vi "SDCP SMF Receiver and Transmitter - Read Processed Trace File.vi"(3 "error in (no error)":errorcluster, 4 "Trace File Path":path=path "E:/Projects/System Diagnostics and Control Protocol/SDCP_LabVIEW/temp/Trace Files/21 Apr 2024 20-17.csv", 5 "Parameter file path":path=path "E:/Projects/System Diagnostics and Control Protocol/SDCP_LabVIEW/Parameter Files/Motion_Processing.param") -> (0 "error out":errorcluster, 1 "Framewise output":cluster{"Data":string[][]}[](array[cluster]), 2 "Output":string[][](array[string]))   [LabVIEW 2020]
uses:
  Typedefs/SDCP - Standard Message Frame Parameters - FGV - commands.ctl
  <vilib>/Utility/file.llb/Read Delimited Spreadsheet (string).vi
  <vilib>/Utility/file.llb/Write Delimited Spreadsheet (string).vi
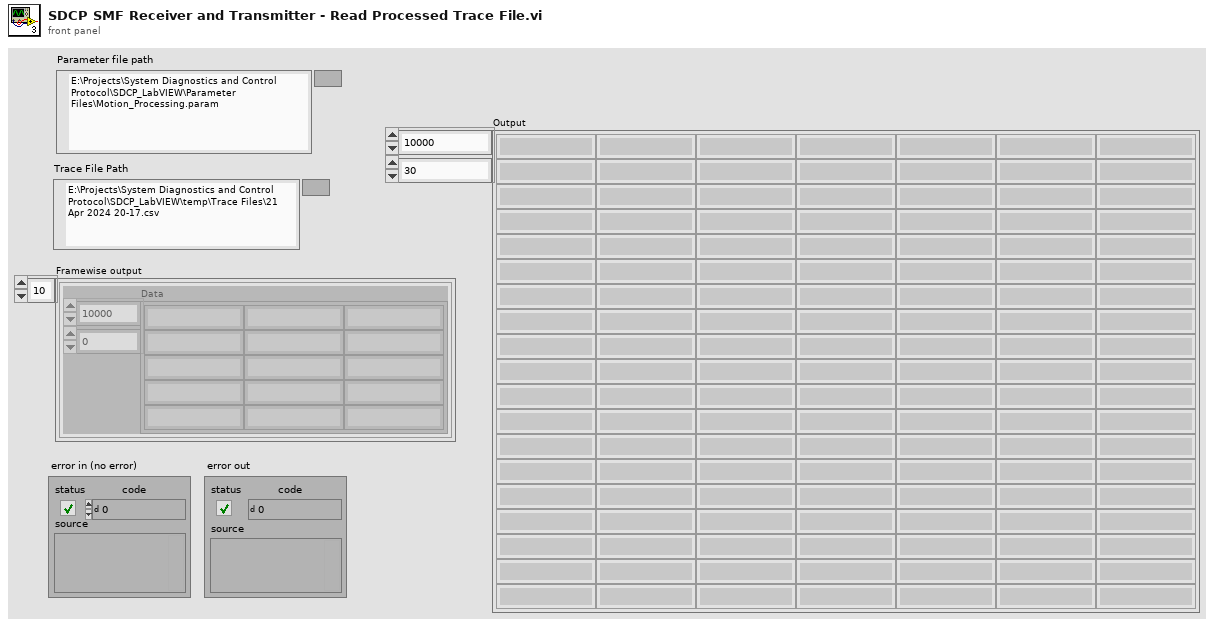
[diagram p1: front panel]
types:
  T1 = cluster{"Data bytes":u8[], "Time (ms)":dbl, "Frame ID":i32}
  T2 = cluster{"Frame ID":i32, "Data":cluster{"Data bytes":u8[], "Time (ms)":dbl}[]}
  T3 = typedef "SDCP - Standard Message Frame Parameters - FGV - commands.ctl" = enum16{"Write descriptors", "Read descriptors", "Read values", "Load parameters from file", "Write values", "Read all descriptors"}
  T4 = typedef "SDCP - SMF parameter descriptors.ctl" = cluster{"Frame name":string, "Frame ID":i32, "Data type":string, "Start Position":i32, "Length":i32, "Factor":dbl, "Offset":dbl, "Parameter name":string, "Value":string}
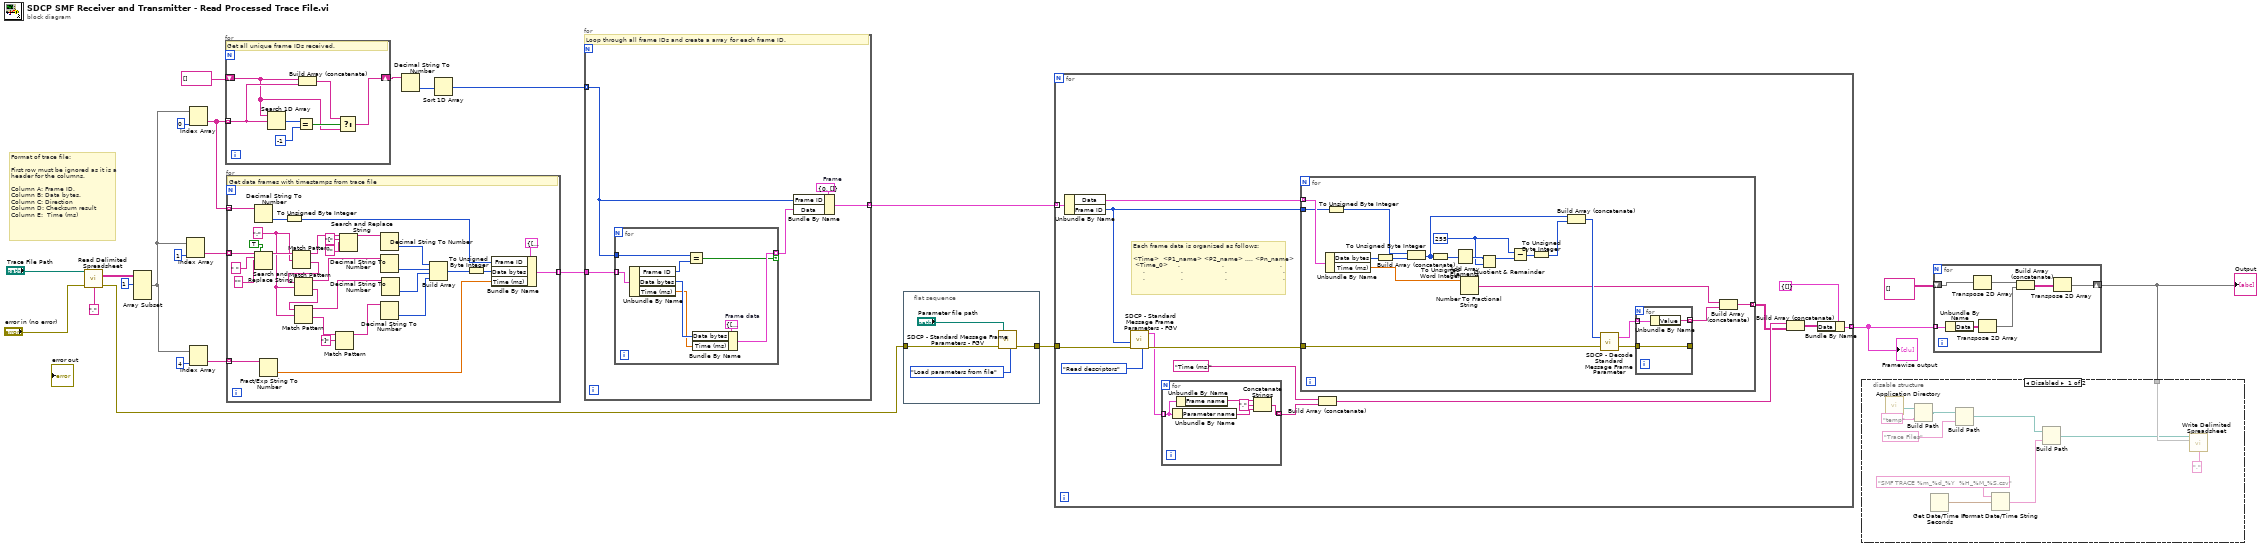
[diagram p0: block diagram]
diagram:
  # "Format of trace file:\n\nFirst row must be ignored as it is a\nheader for the columns.\n\nColumn A: Frame ID.\nColumn B: Data bytes.\nColumn C: Direction\nColumn D: Checksum result\nColumn E:  Time (ms)"
  n1 = call-poly <vilib>:"Read Delimited Spreadsheet.vi"("file path (dialog if empty)"="Trace File Path", "error in (no error)"="error in (no error)", "delimiter (\\t)"="," ("delimiter (\\t)")) -> ("all rows"=w19:string[][], "error out"=w6:errorcluster)  [unwired: 7 in, 4 out]
  n2 = Array Subset(array=w19, index (row)=1 ("index")) -> (w12:string[][])  [unwired: 3 in]
  n3 = Index Array(array=w12, index (col)=1 ("disabled index (col)")) -> (element=w13:string[])  [unwired: 1 in]
  n4 = Index Array(array=w12, index (col)=4 ("disabled index (col)")) -> (element=w10:string[])  [unwired: 1 in]
  n5 = Index Array(array=w12, index (col)=0 ("disabled index (col)")) -> (element=w9:string[])  [unwired: 1 in]
  n6 = for {
    tunnel: w9 -> [w27] mode=indexing
    shift-right: [w24] -> w16
    shift-left: string[] [] -> [w25]
    # "Get all unique frame IDs received."
    n7 = Search 1D Array(1D array=w25, element=w27) -> (index of element=w30:i32)  [unwired: 1 in]
    n8 = Equal?(x=w30, y=-1) -> (x = y?=w28:bool)
    n9 = Build Array (concatenate)(w25, w27) -> (w26:string[])
    n10 = Select(t=w26, s=w28, f=w25) -> (s? t:f=w24:string[])
  }
  n11 = for {
    tunnel: w13 -> [w40] mode=indexing
    tunnel: w10 -> [w36] mode=indexing
    tunnel: [w34] -> w7 mode=indexing
    tunnel: w9 -> [w33] mode=indexing
    w44 = ":" ("regular expression")
    # "Get data frames with timestamps from trace file"
    n12 = Decimal String To Number(string=w33) -> (number=w32:i32)  [unwired: 2 in, 1 out]
    n13 = Search and Replace String(replace all?=TRUE ("replace all? (F)"), input string=w40, search string=" ", replace string="" ("replace string (\"\")")) -> (result string=w48:string)  [unwired: 4 in, 3 out]
    n14 = Fract/Exp String To Number(string=w36) -> (number=w35:dbl)  [unwired: 3 in, 1 out]
    n15 = To Unsigned Byte Integer(number=w32) -> (unsigned 8bit integer=w31:u8)
    n16 = Match Pattern(string=w48, regular expression=w44) -> (before substring=w59:string, after substring=w49:string)  [unwired: 1 in, 2 out]
    n17 = Match Pattern(string=w49, regular expression=w44) -> (before substring=w52:string, after substring=w50:string)  [unwired: 1 in, 2 out]
    n18 = Match Pattern(string=w50, regular expression=w44) -> (before substring=w53:string, after substring=w51:string)  [unwired: 1 in, 2 out]
    n19 = Match Pattern(string=w51, regular expression="]") -> (before substring=w54:string)  [unwired: 1 in, 3 out]
    n20 = Search and Replace String(input string=w59, search string="[", replace string="" ("replace string (\"\")")) -> (result string=w60:string)  [unwired: 5 in, 3 out]
    n21 = Decimal String To Number(string=w60) -> (number=w55:i32)  [unwired: 2 in, 1 out]
    n22 = Decimal String To Number(string=w52) -> (number=w56:i32)  [unwired: 2 in, 1 out]
    n23 = Decimal String To Number(string=w54) -> (number=w58:i32)  [unwired: 2 in, 1 out]
    n24 = Decimal String To Number(string=w53) -> (number=w57:i32)  [unwired: 2 in, 1 out]
    n25 = Build Array(w55, w56, w57, w58) -> (w38:i32[])
    n26 = To Unsigned Byte Integer(number=w38) -> (unsigned 8bit integer=w37:u8[])
    n27 = Bundle By Name(cluster=T1 {"Data bytes"=[], "Time (ms)"=0.0, "Frame ID"=0}, "Frame ID"=w31, "Data bytes"=w37, "Time (ms)"=w35) -> (w34:T1)
  }
  n28 = Decimal String To Number(string=w16) -> (number=w15:i32[])  [unwired: 2 in, 1 out]
  n29 = Sort 1D Array(array=w15) -> (sorted array=w8:i32[])
  n30 = for {
    tunnel: w8 -> [w63] mode=indexing
    tunnel: w7 -> [w65]
    tunnel: [w61] -> w4 mode=indexing
    w64 = T2 {"Frame ID"=0, "Data"=[]}  # Frame
    # "Loop through all frame IDs and create a array for each frame ID."
    n31 = for {
      tunnel: w65 -> [w71] mode=indexing
      tunnel: w63 -> [w72]
      tunnel: [w67] -> w62 mode=indexing if=w66
      w70 = cluster{"Data bytes":u8[], "Time (ms)":dbl} {"Data bytes"=[], "Time (ms)"=0.0}  # Frame data
      n32 = Unbundle By Name(w71) -> ("Frame ID"=w73:i32, "Data bytes"=w69:u8[], "Time (ms)"=w68:dbl)
      n33 = Equal?(x=w72, y=w73) -> (x = y?=w66:bool)
      n34 = Bundle By Name(cluster=w70, "Data bytes"=w69, "Time (ms)"=w68) -> (w67:cluster{"Data bytes":u8[], "Time (ms)":dbl})
    }
    n35 = Bundle By Name(cluster=w64, "Frame ID"=w63, "Data"=w62) -> (w61:T2)
  }
  n36 = flat-sequence {
    tunnel: w6 -> [w77]
    tunnel: [w74] -> w5
    frame #0 {
      n37 = call "SDCP - Standard Message Frame Parameters - FGV.vi"("Parameter file path"="Parameter file path", "error in (no error)"=w77, "Command"=SDCP_-_Standard_Message_Frame_Parameters_-_FGV_-_commands."Load parameters from file") -> ("error out"=w74:errorcluster)  [unwired: 4 in, 1 out]
    }
  }
  n38 = for {
    tunnel: w5 -> [w89]
    tunnel: w4 -> [w91] mode=indexing
    tunnel: [w78] -> w1 mode=indexing
    # "Each frame data is organized as follows:\n\n<Time>  <P1_name> <P2_name> .... <Pn_name>\n <Time_0>     .                     .                            .\n     .                  .                     .                            .\n     .                  .                     .                            ."
    n39 = Unbundle By Name(w91) -> ("Data"=w90:cluster{"Data bytes":u8[], "Time (ms)":dbl}[], "Frame ID"=w86:i32)
    n40 = call "SDCP - Standard Message Frame Parameters - FGV.vi"("FID"=w86, "error in (no error)"=w89, "Command"=SDCP_-_Standard_Message_Frame_Parameters_-_FGV_-_commands."Read descriptors") -> ("SMF Parameters descriptors out"=w85:T4[], "error out"=w88:errorcluster)  [unwired: 4 in]
    n41 = for {
      tunnel: w85 -> [w96] mode=indexing
      tunnel: [w95] -> w84 mode=indexing
      n42 = Unbundle By Name(w96) -> ("Parameter name"=w92:string)
      n43 = Unbundle By Name(w96) -> ("Frame name"=w94:string)
      n44 = Concatenate Strings(w94, "." ("string"), w92) -> (w95:string)
    }
    n45 = for {
      tunnel: w90 -> [w116] mode=indexing
      tunnel: w88 -> [w115]
      tunnel: w86 -> [w113]
      tunnel: [w97] -> w81 mode=indexing
      w108 = u16 255 ("x")
      n46 = Unbundle By Name(w116) -> ("Data bytes"=w114:u8[], "Time (ms)"=w99:dbl)
      n47 = To Unsigned Byte Integer(number=w113) -> (unsigned 8bit integer=w104:u8)
      n48 = To Unsigned Byte Integer(number=w114) -> (unsigned 8bit integer=w105:u8[])
      n49 = Build Array (concatenate)(w104, w105) -> (w107:u8[])
      n50 = To Unsigned Word Integer(number=w107) -> (unsigned 16bit integer=w112:u16[])
      n51 = Add Array Elements(numeric array=w112) -> (sum=w109:u16)
      n52 = Number To Fractional String(number=w99) -> (F-format string=w98:string)  [unwired: 3 in]
      n53 = Quotient & Remainder(x=w109, y=w108) -> (x-y*floor(x/y)=w111:u16)  [unwired: 1 out]
      n54 = Subtract(x=w108, y=w111) -> (x-y=w110:u16)
      n55 = To Unsigned Byte Integer(number=w110) -> (unsigned 8bit integer=w106:u8)
      n56 = Build Array (concatenate)(w107, w106) -> (w103:u8[])
      n57 = call "SDCP - Decode Standard Message Frame Parameter.vi"("error in (no error)"=w115, "Bytes in"=w103) -> ("error out"=w101:errorcluster, "SMF Parameters out"=w102:T4[])
      n58 = for {
        tunnel: w102 -> [w119] mode=indexing
        tunnel: w101 -> [w118]
        tunnel: [w118] -> _
        tunnel: [w117] -> w100 mode=indexing
        n59 = Unbundle By Name(w119) -> ("Value"=w117:string)
      }
      n60 = Build Array (concatenate)(w98, w100) -> (w97:string[])
    }
    n61 = Build Array (concatenate)("Time (ms)", w84) -> (w82:string[])
    n62 = Build Array (concatenate)(w82, w81) -> (w79:string[][])
    n63 = Bundle By Name(cluster=cluster{"Data":string[][]} {"Data"=[]}, "Data"=w79) -> (w78:cluster{"Data":string[][]})
  }
  "Framewise output" <- w1
  n64 = for {
    tunnel: w1 -> [w125] mode=indexing
    shift-right: [w120] -> w2
    shift-left: string[][] [] -> [w126]
    n65 = Unbundle By Name(w125) -> ("Data"=w124:string[][])
    n66 = Transpose 2D Array(2D array=w126) -> (transposed array=w121:string[][])
    n67 = Transpose 2D Array(2D array=w124) -> (transposed array=w122:string[][])
    n68 = Build Array (concatenate)(w121, w122) -> (w123:string[][])
    n69 = Transpose 2D Array(2D array=w123) -> (transposed array=w120:string[][])
  }
  "Output" <- w2
  n70 = disable-structure shown="Disabled" {
    disable-tunnel: w2 -> [w137 _]
    frame Disabled {
      n71 = call <vilib>:"Application Directory.vi"() -> ("Application Directory"=w133:path)
      n72 = Build Path(base path=w133, name or relative path="temp") -> (appended path=w131:path)
      n73 = Get Date/Time In Seconds() -> (seconds since 1Jan1904=w135:timestamp)
      n74 = Build Path(base path=w131, name or relative path="Trace Files") -> (appended path=w129:path)
      n75 = Format Date/Time String(time format string (%c)="SMF TRACE %m_%d_%Y  %H_%M_%S.csv", seconds (now)=w135) -> (date/time string=w128:string)  [unwired: 1 in]
      n76 = Build Path(base path=w129, name or relative path=w128) -> (appended path=w127:path)
      n77 = call-poly <vilib>:"Write Delimited Spreadsheet.vi"("file path (dialog if empty)"=w127, "2D data"=w137, "delimiter (\\t)"="," ("delimiter (\\t)")) -> ()  [unwired: 11 in, 2 out]
    }
    frame Enabled {
    }
  }
